vi "GlobalMenuReference.vi"() -> ()   [LabVIEW 2012]
panel:
  in  "Menu Refnum":refnum<k9>
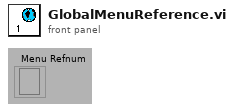
[diagram p1: front panel]
diagram:
